vi "Read Teller.vi"(11 "Stop Msg in":refnum<class "--Stop Msg.lvclass">) -> (2 "Teller":refnum<class "Teller.lvclass">)   [LabVIEW 2025, in "jettl.lvlib" / "Stop jettl Msg.lvlib" / "--Stop Msg.lvclass"]
uses:
  --Stop Msg.lvclass
  Teller/Teller.lvclass
  --Stop Msg.lvclass/--Stop Msg.ctl
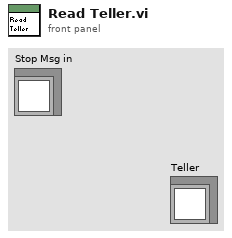
[diagram p1: front panel]
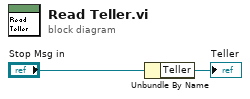
[diagram p0: block diagram]
diagram:
  n1 = Unbundle By Name("Stop Msg in") -> ("Teller"=→"Teller":refnum<class "Teller.lvclass">)
